vi "extract ROI image.vi"(4 "NO.":i32, 6 "snapshot NO.":i32, 9 "beads track":T1[](array[typedef]) {"centroid"."Y Centroid" format="%.2f"; "centroid"."X Centroid" format="%.2f"; "ROI Des out"."Contours"."Type" items=["No Selection", "Point", "Line", "Rectangle", "Oval", "Polygon", "Freehand Region", "Annulus", "Unused2", "Unused3", "Broken Line", "Freehand Line", "Rotated Rectangle"]}, 10 "CCD image":T3[](array[typedef])) -> (2 "Image Out":T3)   [LabVIEW 2017]
uses:
  <vilib>/vision/Image Controls.llb/IMAQ Image.ctl
  control/Bead track.ctl
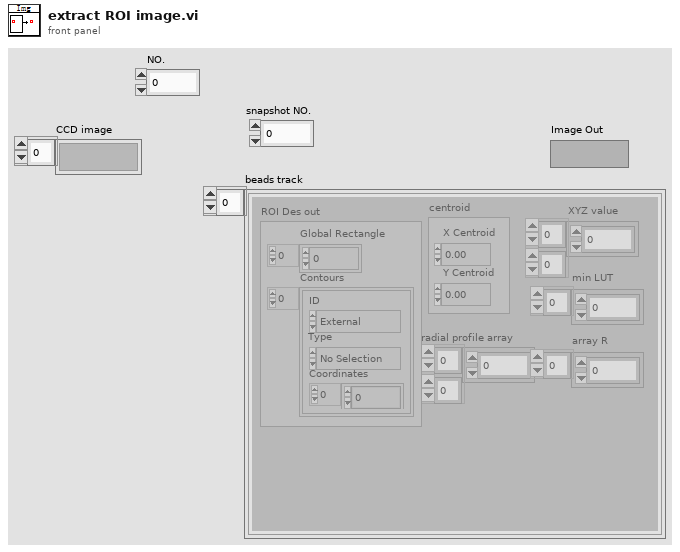
[diagram p1: front panel]
types:
  T1 = typedef "Bead track.ctl" = cluster{"XYZ value":dbl[][], "radial profile array":dbl[][], "min LUT":dbl[], "ROI Des out":T2, "array R":dbl[], "centroid":cluster{"X Centroid":sgl, "Y Centroid":sgl}}
  T2 = typedef "ROI Descriptor" = cluster{"Global Rectangle":i32[], "Contours":cluster{"ID":enum32{"External", "Internal"}, "Type":u32, "Coordinates":i32[]}[]}
  T3 = typedef "IMAQ Image.ctl" = refnum<image>
  T4 = typedef "IMAQ Rectangle" = cluster{"Left":i32, "Top":i32, "Right":i32, "Bottom":i32, "Rotation":dbl}
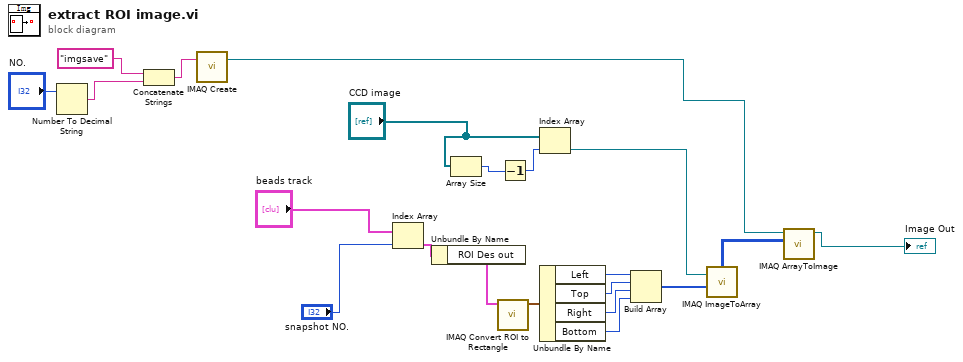
[diagram p0: block diagram]
diagram:
  n1 = Number To Decimal String(number="NO.") -> (decimal integer string=w4:string)  [unwired: 1 in]
  n2 = Concatenate Strings("imgsave" ("string"), w4) -> (w2:string)
  n3 = call "IMAQ Create"("Image Name"=w2) -> ("New Image"=w5:T3)  [unwired: 4 in, 1 out]
  n4 = Index Array(array="beads track", index="snapshot NO.") -> (element=w16:T1)
  n5 = Unbundle By Name(w16) -> ("ROI Des out"=w10:T2)
  n6 = Array Size(array="CCD image") -> (size(s)=w19:i32)
  n7 = call "IMAQ Convert ROI to Rectangle"("ROI Descriptor"=w10) -> ("Rectangle"=w11:T4)  [unwired: 8 in, 1 out]
  n8 = Decrement(x=w19) -> (x-1=w18:i32)
  n9 = Index Array(array="CCD image", index=w18) -> (element=w8:T3)
  n10 = Unbundle By Name(w11) -> ("Left"=w15:i32, "Top"=w13:i32, "Right"=w14:i32, "Bottom"=w12:i32)
  n11 = Build Array(w15, w13, w14, w12) -> (w9:i32[])
  n12 = call "IMAQ ImageToArray"("Optional Rectangle"=w9, "Image"=w8) -> ("Image Pixels (U8)"=w7:u8[][])  [unwired: 2 in, 4 out]
  n13 = call "IMAQ ArrayToImage"("Image Pixels (U8)"=w7, "Image"=w5) -> ("Image Out"=→"Image Out":T3)  [unwired: 8 in, 1 out]
